vi "file exists.vi"(11 "Path in":path) -> (2 "file exists":bool, 3 "Path out":path)   [LabVIEW 2013]
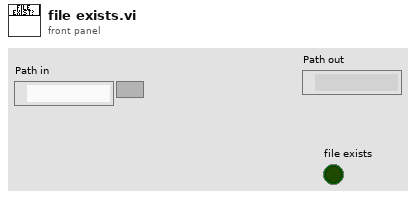
[diagram p1: front panel]
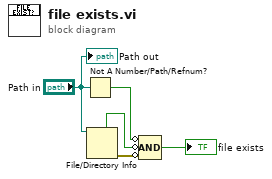
[diagram p0: block diagram]
diagram:
  n1 = Not A Number/Path/Refnum?(number/path/refnum="Path in") -> (NaN/Path/Refnum?=w4:bool)
  n2 = File/Directory Info(path="Path in") -> (directory=w3:bool, error out=w2:errorcluster)  [unwired: 1 in, 5 out]
  n3 = Compound Arithmetic op=AND(invert w4, invert w3, invert w2) -> (→"file exists":bool)
  "Path out" <- "Path in"
